vi "calculateTimeStep.vi"(8 "error in (no error)":errorcluster, 11 "RampAction in":refnum<class "RampAction.lvclass">) -> (0 "error out":errorcluster, 3 "RampAction out":refnum<class "RampAction.lvclass">)   [LabVIEW 2011, in "Views.lvlib" / "ScriptEditor.lvlib" / "RampAction.lvclass"]
uses:
  RampAction.lvclass
  RampAction.lvclass/RampAction.ctl
  ActionPanel.lvclass
  Tools/Scripting/ScriptingEvent/ScriptEvents/Ramp/RampEvent/RampEvent.lvclass
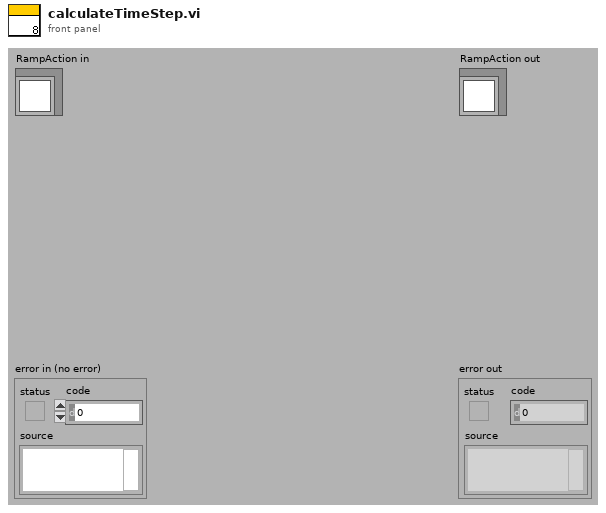
[diagram p1: front panel]
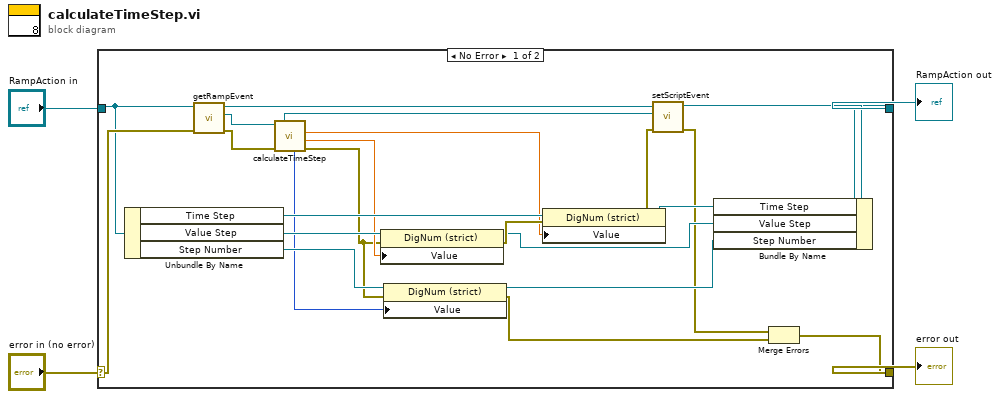
[diagram p0: block diagram]
diagram:
  n1 = case shown="No Error" "error in (no error)" {
    selector: "error in (no error)" -> [w26 w29]
    tunnel: [w5 w29] -> w3
    tunnel: [w12 w28] -> w1
    tunnel: "RampAction in" -> [w22 w28]
    frame No Error {
      n2 = Unbundle By Name(w22) -> ("Time Step"=w21:refnum<vi>, "Value Step"=w19:refnum<vi>, "Step Number"=w11:refnum<vi>)
      n3 = call "getRampEvent.vi"("error in (no error)"=w26, "RampAction in"=w22) -> ("error out"=w24:errorcluster, "RampEvent"=w25:refnum<class "RampEvent.lvclass">, "RampAction out"=w27:refnum<class "RampAction.lvclass">)  [unwired: 7 in]
      n4 = call "calculateTimeStep.vi"("error in (no error)"=w24, "RampEvent in"=w25) -> ("error out"=w10:errorcluster, "valueStep"=w18:dbl, "timeStep"=w17:dbl, "RampEvent out"=w23:refnum<class "RampEvent.lvclass">, "number of Steps"=w9:i32)  [unwired: 5 in]
      n5 = property class="DigNum (strict)"(reference=w19, error in=w10, "Value"=w18) -> (reference out=w14:refnum<vi>, error out=w20:errorcluster)
      n6 = property class="DigNum (strict)"(reference=w11, error in=w10, "Value"=w9) -> (reference out=w8:refnum<vi>, error out=w6:errorcluster)
      n7 = property class="DigNum (strict)"(reference=w21, error in=w20, "Value"=w17) -> (reference out=w15:refnum<vi>, error out=w16:errorcluster)
      n8 = call "setScriptEvent.vi"("error in (no error)"=w16, "ScriptEvent.lvclass"=w23, "ActionPanel.lvclass in"=w27) -> ("error out"=w7:errorcluster, "ActionPanel.lvclass out"=w13:refnum<class "RampAction.lvclass">)  [unwired: 7 in]
      n9 = Bundle By Name(cluster=w13, "Time Step"=w15, "Value Step"=w14, "Step Number"=w8) -> (w12:refnum<class "RampAction.lvclass">)
      n10 = Merge Errors(w7, w6) -> (w5:errorcluster)
    }
    frame Error {
    }
  }
  "error out" <- w3
  "RampAction out" <- w1
